vi "Measurement Logic.vi"() -> ()   [LabVIEW 2021, in "Game Of Life.lvlib"]
uses:
  Game Of Life.lvlib
  Measurement Configuration.ctl
  Measurement Results.ctl
  <vilib>/gRPC/Generated APIs/ni/protobuf/types/RPC Messages/ni_protobuf_types_DoubleXYData.ctl
  <vilib>/Plug-In SDKs/Measurements/Measure Call Context/Measure Call Context.lvclass
  <vilib>/numeric/Random Number (Range) U64.vi
  <vilib>/numeric/sub_Random U32.vi
  <vilib>/gRPC/Generated APIs/ni/protobuf/types/ni.protobuf.types.lvlib
panel:
  out "measure call context out":refnum<class "Measure Call Context.lvclass">
  in  "measure call context in":refnum<class "Measure Call Context.lvclass">
  out "measurement results":T1
  in  "measurement configuration":T3
  out "error out":errorcluster
  in  "error in":errorcluster
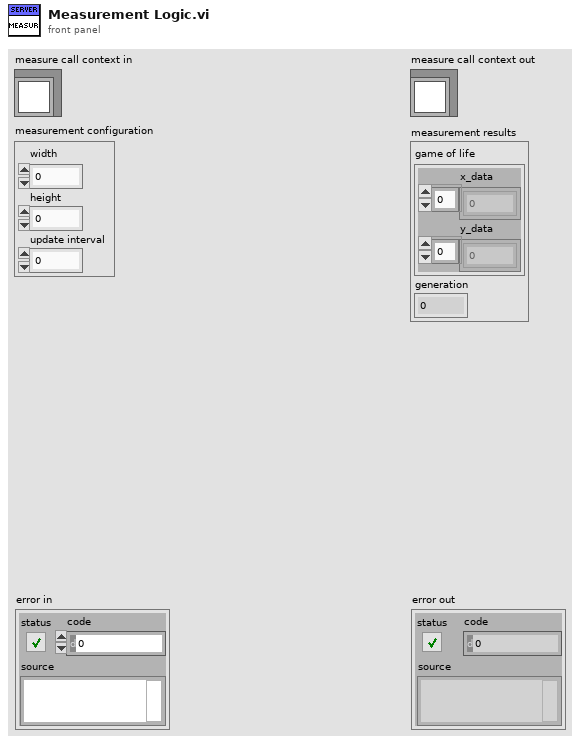
[diagram p1: front panel]
types:
  T1 = typedef "Game Of Life.lvlib/Measurement Results.ctl" = cluster{"game of life":T2, "generation":u32}
  T2 = typedef "ni.protobuf.types.lvlib/ni_protobuf_types_DoubleXYData.ctl" = cluster{"x_data":dbl[], "y_data":dbl[]}
  T3 = typedef "Game Of Life.lvlib/Measurement Configuration.ctl" = cluster{"width":u32, "height":u32, "update interval":u32}
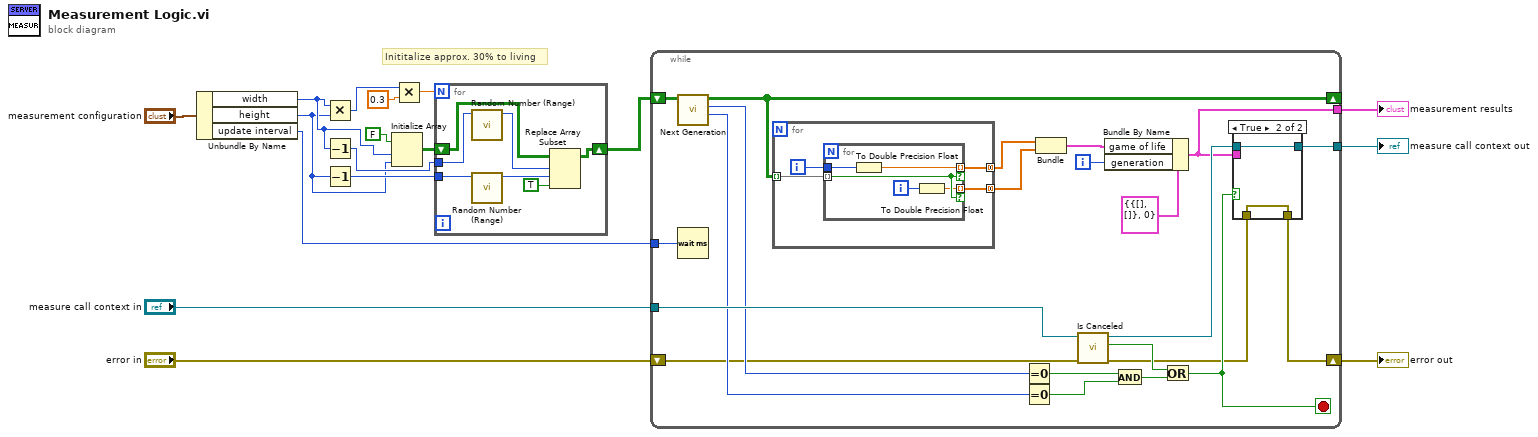
[diagram p0: block diagram]
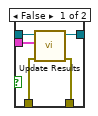
[diagram p2: hidden frame]
diagram:
  # "Inititalize approx. 30% to living"
  n1 = Unbundle By Name("measurement configuration") -> ("width"=w8:u32, "height"=w7:u32, "update interval"=w13:u32)
  n2 = Multiply(x=w8, y=w7) -> (x*y=w6:u32)
  n3 = Decrement(x=w8) -> (x-1=w11:u32)
  n4 = Decrement(x=w7) -> (x-1=w10:u32)
  n5 = Initialize Array(FALSE, w8, w7) -> (w9:bool[][])
  n6 = Multiply(x=w6, y=0.3) -> (x*y=w4:dbl)
  n7 = for {
    N: w4 -> [_]
    tunnel: w11 -> [w24]
    tunnel: w10 -> [w23]
    shift-right: [w18] -> w3
    shift-left: w9 -> [w22]
    n8 = call-poly <vilib>:"Random Number (Range).vi"("upper bound (100)"=w24) -> ("number"=w21:u64)  [unwired: 10 in]
    n9 = call-poly <vilib>:"Random Number (Range).vi"("upper bound (100)"=w23) -> ("number"=w20:u64)  [unwired: 10 in]
    n10 = Replace Array Subset(array=w22, new element=TRUE ("new element/subarray"), index (row)=w21, index (col)=w20) -> (w18:bool[][])
  }
  n11 = while {
    shift-right: [w39] -> _
    shift-left: w3 -> [w46]
    tunnel: "measure call context in" -> [w44]
    tunnel: [w42] -> w15
    tunnel: [w40] -> w14
    tunnel: w13 -> [w37]
    shift-right: [w31] -> w1
    shift-left: "error in" -> [w28]
    i -> [w38]
    stop <- w36 stop-if-true
    n12 = call "Next Generation.vi"("cells in"=w46) -> ("deaths"=w34:i32, "births"=w35:i32, "cells out"=w39:bool[][])  [unwired: 8 in]
    n13 = Wait (ms)(milliseconds to wait=w37) -> ()  [unwired: 1 out]
    n14 = for {
      tunnel: w39 -> [w50] mode=indexing
      tunnel: [w48] -> w25 mode=concatenating
      tunnel: [w47] -> w26 mode=concatenating
      i -> [w49]
      n15 = for {
        tunnel: w50 -> [w55] mode=indexing
        tunnel: [w53] -> w48 mode=indexing if=w55
        tunnel: w49 -> [w54]
        tunnel: [w51] -> w47 mode=indexing if=w55
        i -> [w52]
        n16 = To Double Precision Float(number=w54) -> (double precision float=w53:dbl)
        n17 = To Double Precision Float(number=w52) -> (double precision float=w51:dbl)
      }
    }
    n18 = Equal To 0?(x=w35) -> (x = 0?=w33:bool)
    n19 = Equal To 0?(x=w34) -> (x = 0?=w32:bool)
    n20 = Bundle(w25, w26) -> (w41:cluster{dbl[], dbl[]})  [unwired: 1 in]
    n21 = call <vilib>:"Is Canceled.vi"("error in"=w28, "measure call context in"=w44) -> ("error out"=w27:errorcluster, "is canceled?"=w29:bool, "measure call context out"=w43:refnum<class "Measure Call Context.lvclass">)  [unwired: 7 in]
    n22 = Bundle By Name(cluster=T1 {"game of life"={"x_data"=[], "y_data"=[]}, "generation"=0} ("Measurement Results"), "game of life"=w41, "generation"=w38) -> (w40:T1)
    n23 = And(x=w33, y=w32) -> (x .and. y?=w30:bool)
    n24 = Or(x=w29, y=w30) -> (x .or. y?=w36:bool)
    n25 = case shown="True" w36 {
      tunnel: w43 -> [w60 w62]
      tunnel: [w59 w62] -> w42
      tunnel: w40 -> [w58 _]
      tunnel: w27 -> [w57 w61]
      tunnel: [w56 w61] -> w31
      frame False {
        n26 = call <vilib>:"Update Results.vi"("error in"=w57, "measurement results"=w58, "measure call context in"=w60) -> ("error out"=w56:errorcluster, "measure call context out"=w59:refnum<class "Measure Call Context.lvclass">)  [unwired: 7 in]
      }
      frame True {
      }
    }
  }
  "error out" <- w1
  "measurement results" <- w14
  "measure call context out" <- w15
